vi "Robot Main.vi"   [LabVIEW 2012]
doc: "This VI imlements the framework and scheduler for your robotics program. It should not be necessary to modify the framework. You are expected to add your code to the VIs called from Robot Main, the ones located in the Team Code within the project."
panel:
  # "2013 Uber Code, FINAL"
  # "Version 2.2_Sat: 3-28-13"
  # "Controls"
  # "PWM"
  # "DIO"
  # "Relay"
  # "Solenoid"
  # "Todo"
  # "Analog"
  # "JS 1\nX Axis: Arcade Drive \nY Axis: Arcade Drive \nZ Axis:\nButton 1: \nButton 2:\nButton 3:\nButton 4:\nButton 5:\nButton 6: Shift High\nButton 7: Hold Position (Toggle)\nButton 8: Stop Tracking\nButton 9: Shift Low\nButton 10:\nButton 11: To Driver Control\nButton 12:"
  # "JS 2\nX Axis: \nY Axis: Shooter Arm\nZ Axis: \nButton 1: Stop Tracking\nButton 2: Hold Positon\nButton 3: Track High\nButton 4: Track Mid Left\nButton 5: Track Mid Right\nButton 6: Feeder Ready\nButton 7: Stop Feeder \nButton 8: Home Shooter Arm\nButton 9: Home Auger\nButton 10: Arm Driver\nButton 11: Arm Manual\nButton 12:"
  # "1 a): Right Front Drive\n1 b): Right Rear Drive\n2 a): Left Front Drive\n2 b): Left Rear Drive\n3 a): Right Shooter Angle\n3 b): Left Shooter Angle\n     4: Shooter Belt\n     5: Rear Shooter \n     6: Front Shooter\n     7: Auger\n     8: \n     9: \n   10:"
  # "1: Right Drive Encoder A\n  2: Right Drive Encoder B\n  3: Left Drive Encoder A  \n  4: Left Drive Encoder B\n  5: Auger Encoder A\n  6: Auger Encoder B\n  7: Shooter Angle Encoder A\n  8: Shooter Angle Encoder B\n  9: Shooter Angle Encoder Index\n10:\n11:\n12:\n13: Auger Light Sensor \n14: Pneumatic Pressure Switch"
  # "1: Compressor Spike\n2:\n3:\n4:\n5:\n6:\n7:\n8:"
  # "1:\n2:\n3:\n4:\n5:\n6:\n7:\n8:"
  # "1: Shifter A\n2: Shifter B\n3: Shooter End A\n4: Shooter End B\n5: Pickup A\n6: Pickup B\n7:\n8:"
  # "JS 3\nX Axis: \nY Axis: Auger (Manual)\nZ Axis: Shooter Speed (Manual)\nButton 1: \nButton 2: Auger Index Up\nButton 3: Auger Index Down\nButton 4: Shooter Belt In\nButton 5:Shooter Belt Out\nButton 6: Enable Auger DC\nButton 7: Disable Auger DC\nButton 8: Disable Auger Manual\nButton 9: Enable Auger Manual\nButton 10: Disable Shooter Manual\nButton 11: Enable Shooter Manual\nButton 12:"
  # "- Make Work\n- Update Vision Values\n   - Color Filters\n   - Target Selection, Scoring\n   - vision data->angle \n- Implement Target Selection\n- Change Auger PID to rate\n- Init frisbee storage array (switch)\n- data logging\n- better auto stucture\n     - auto files (VALIDATE!!!)"
  # "Revision History"
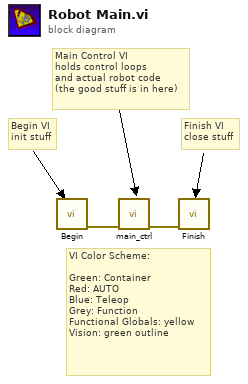
[diagram p0: block diagram]
diagram:
  # "Finish VI\nclose stuff"
  # "Main Control VI\nholds control loops\nand actual robot code\n(the good stuff is in here)"
  # "Begin VI\ninit stuff"
  # "VI Color Scheme:\n\nGreen: Container\nRed: AUTO\nBlue: Teleop\nGrey: Function\nFunctional Globals: yellow\nVision: green outline"
  n1 = call "Begin.vi"() -> ("error out"=w2:errorcluster)  [unwired: 1 in, 10 out]
  n2 = call "main_ctrl.vi"("error in"=w2) -> ("error out"=w1:errorcluster)  [unwired: 10 in]
  n3 = call "Finish.vi"("error in"=w1) -> ()  [unwired: 7 in]
